vi "Robo Drive.vi"(6 "Button Flip Directions":bool, 8 "Right Analog (axes 3)":dbl, 9 "Left Analog (axes 2)":dbl, 10 "Axes 1 (y axis)":dbl, 11 "Axes 0 (x axis)":dbl) -> ()   [LabVIEW 2014]
uses:
  <vilib>/Rock Robotics/WPI/RobotDrive/WPI_RobotDriveGetSetRefNum.vi
  <vilib>/Rock Robotics/Network Tables/SD Write Numeric Array.vi
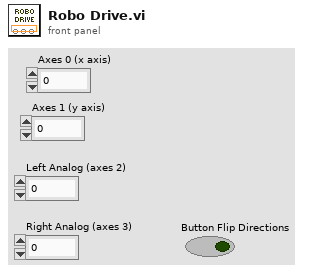
[diagram p1: front panel]
types:
  T1 = typedef "WPI_RobotDriveDevRef.ctl" = cluster{"DevStatus":errorcluster, "Motors[]":T2[], "Square Inputs":bool, "Max Output":dbl}
  T2 = typedef "WPI_MotorControlDeviceRef.ctl" = cluster{"DeviceStatus":errorcluster, "Type":T3, "PWM":cluster{"Controller":T4, "PWM Channel":T5, "DeadBand":T6}, "CAN":cluster{"Device Number":u8, "Control Mode":T7, "Semaphore":T8, "Max Vout":dbl, "TalonSRX Control Mode":T9}, "Invert":bool, "TransformRef":T10, "InvTransformRef":T10}
  T3 = typedef "WPI_MotorControlType.ctl" = enum16{"PWM", "CAN", "CANTalonSRX"}
  T4 = typedef "FPGA_TypedefDigitalModule.ctl" = enum16{"Controller 1"}
  T5 = typedef "FPGA_DIOPWMChannel.ctl" = enum8{"PWM 0", "PWM 1", "PWM 2", "PWM 3", "PWM 4", "PWM 5", "PWM 6", "PWM 7", "PWM 8", "PWM 9", "PWM MXP 0", "PWM MXP 1", "PWM MXP 2", "PWM MXP 3", "PWM MXP 4", "PWM MXP 5", "PWM MXP 6", "PWM MXP 7", "PWM MXP 8", "PWM MXP 9", "Invalid"}
  T6 = typedef "WPI_PWMDeadband.ctl" = cluster{"Name":string, "maxPositivePwm":i32, "minPositivePwm":i32, "centerPwm":i32, "maxNegativePwm":i32, "minNegativePwm":i32, "angularRange":u16}
  T7 = typedef "WPI_CANJaguar_ControlMode.ctl" = enum8{"Percent VBus", "Current", "Speed", "Position", "Voltage"}
  T8 = typedef "Semaphore RefNum" = refnum<k1>
  T9 = typedef "WPI_CANTalonSRX_APIControlMode.ctl" = enum8{"Percent VBus", "Speed", "Position", "Slave", "Unchanged / Invalid"}
  T10 = typedef "WPI_PWMTransform_ConPane.ctl" = refnum<vi>
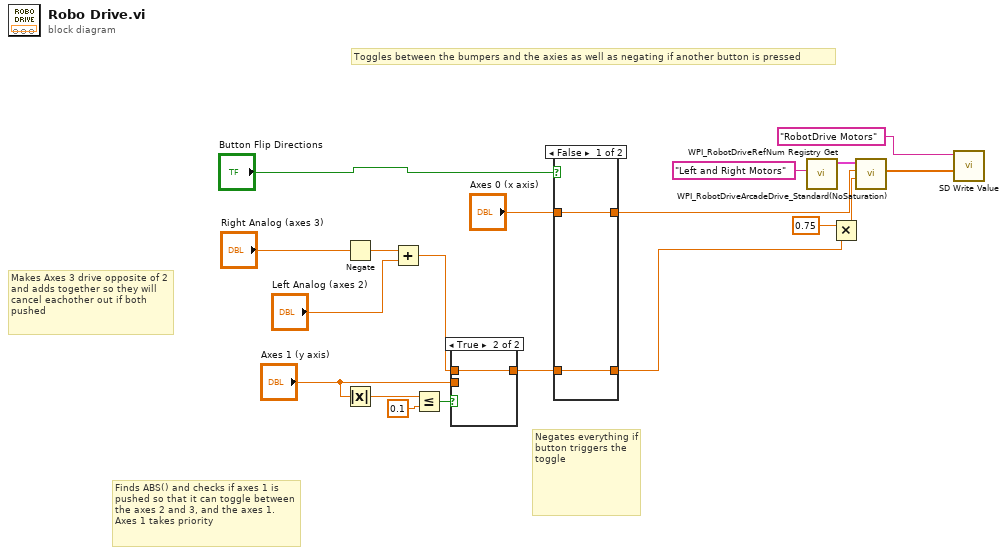
[diagram p0: block diagram]
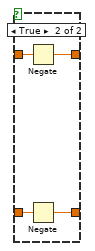
[diagram p2: hidden frame]
diagram:
  # "Toggles between the bumpers and the axies as well as negating if another button is pressed"
  # "Negates everything if button triggers the toggle"
  # "Finds ABS() and checks if axes 1 is pushed so that it can toggle between the axes 2 and 3, and the axes 1. Axes 1 takes priority"
  # "Makes Axes 3 drive opposite of 2 and adds together so they will cancel eachother out if both pushed"
  n1 = Negate(x="Right Analog (axes 3)") -> (-x=w10:dbl)
  n2 = Absolute Value(x="Axes 1 (y axis)") -> (abs(x)=w16:dbl)
  n3 = Add(x=w10, y="Left Analog (axes 2)") -> (x+y=w17:dbl)
  n4 = Less Or Equal?(x=w16, y=0.1) -> (x <= y?=w18:bool)
  n5 = case shown="True" w18 {
    tunnel: "Axes 1 (y axis)" -> [w20 _]
    tunnel: w17 -> [_ w21]
    tunnel: [w20 w21] -> w15
    frame False {
    }
    frame True {
    }
  }
  n6 = case shown="False" "Button Flip Directions" {
    tunnel: w15 -> [w22 w27]
    tunnel: "Axes 0 (x axis)" -> [w23 w26]
    tunnel: [w23 w25] -> w5
    tunnel: [w22 w24] -> w4
    frame False {
    }
    frame True {
      n7 = Negate(x=w26) -> (-x=w25:dbl)
      n8 = Negate(x=w27) -> (-x=w24:dbl)
    }
  }
  n9 = call <vilib>:"WPI_RobotDriveRefNum Registry Get.vi"("refnum name"="Left and Right Motors") -> ("RobotDriveDevRef"=w6:T1)  [unwired: 1 in, 9 out]
  n10 = Multiply(x=0.75, y=w4) -> (x*y=w3:dbl)
  n11 = call <vilib>:"WPI_RobotDriveArcadeDrive_Standard(NoSaturation).vi"("Y axis value"=w3, "X axis value"=w5, "RobotDriveDevRef"=w6) -> ("Motor Values"=w7:dbl[])  [unwired: 1 in, 7 out]
  n12 = call-poly <vilib>:"SD Write Value.vi"("Numeric Array"=w7, "Name"="RobotDrive Motors") -> ()  [unwired: 8 in, 2 out]
